vi "Request Target Connections.vi"(8 "error in":errorcluster) -> (0 "error out":errorcluster)   [LabVIEW 2021, in "Host Interpreter.lvlib"]
uses:
  Host Interpreter.lvlib
  Libraries/UDP Comms/UDP Message--cluster.ctl
  Libraries/UDP Comms/UDP Comms.lvlib
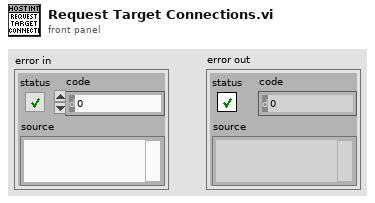
[diagram p1: front panel]
types:
  T1 = typedef "UDP Comms.lvlib/UDP Message--cluster.ctl" = cluster{"Command":string, "Data":variant}
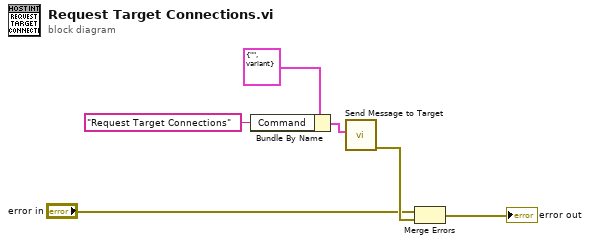
[diagram p0: block diagram]
diagram:
  n1 = Bundle By Name(cluster=T1 {"Command"="", "Data"=variant} ("UDP Message--cluster"), "Command"="Request Target Connections") -> (w6:T1)
  n2 = call "Send Message to Target.vi"("UDP Message--cluster"=w6) -> ("error out"=w3:errorcluster)  [unwired: 10 in]
  n3 = Merge Errors("error in", w3) -> (→"error out":errorcluster)
